vi "CommonVIs_UmlOpenVIRef.vi"(6 "ProjectNameIn":string, 8 "error in":errorcluster, 10 "ViPath/ViName":variant, 11 "AppRef":refnum<vi>) -> (0 "error out":errorcluster, 3 "vi reference":refnum<vi>, 4 "ProjectNameOut":string, 5 "AppRefOut":refnum<vi>)   [LabVIEW 2020]
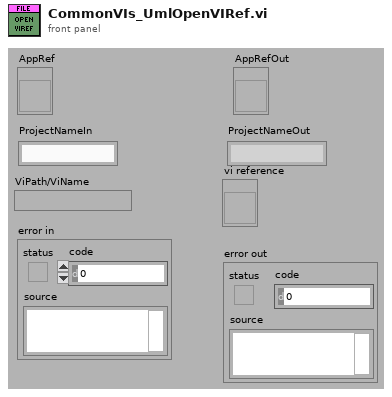
[diagram p1: front panel]
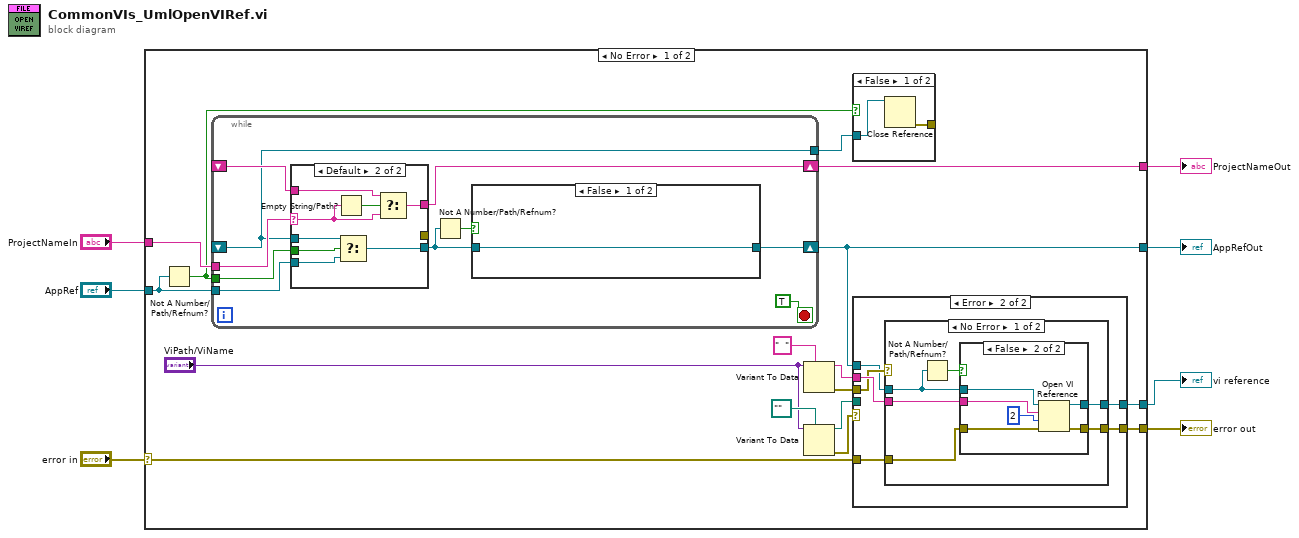
[diagram p0: block diagram]
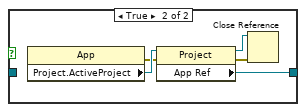
[diagram p3: hidden frame]
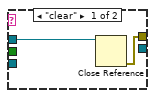
[diagram p4: hidden frame]
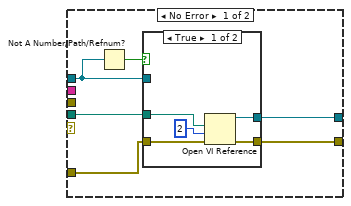
[diagram p5: hidden frame]
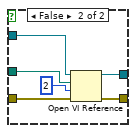
[diagram p6: hidden frame]
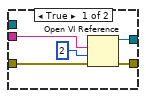
[diagram p7: hidden frame]
diagram:
  n1 = case shown="No Error" "error in" {
    selector: "error in" -> [w15 w93]
    tunnel: [w23 w93] -> w7
    tunnel: [w22 _] -> w6
    tunnel: "AppRef" -> [w10 _]
    tunnel: [w13 _] -> w3
    tunnel: "ProjectNameIn" -> [w12 _]
    tunnel: [w11 _] -> w1
    frame No Error {
      n2 = Not A Number/Path/Refnum?(number/path/refnum=w10) -> (NaN/Path/Refnum?=w9:bool)
      n3 = while {
        shift-right: [w26] -> w13
        shift-left: _ -> [w29]
        tunnel: w10 -> [w34]
        shift-right: [w32] -> w11
        shift-left: _ -> [w33]
        tunnel: w12 -> [w30]
        tunnel: w9 -> [w31]
        tunnel: [w29] -> w8
        stop <- TRUE stop-if-true
        n4 = case shown="Default" w30 {
          selector: w30 -> [_ w44]
          tunnel: w34 -> [_ w51]
          tunnel: [_ w50] -> w27
          tunnel: w33 -> [_ w49]
          tunnel: [_ w48] -> w32
          tunnel: w31 -> [_ w47]
          tunnel: w29 -> [w43 w46]
          tunnel: [w42 _] -> _
          frame "clear" {
            n5 = Close Reference(reference=w43) -> (error out=w42:errorcluster)  [unwired: 1 in]
          }
          frame Default {
            n6 = Empty String/Path?(string/path=w44) -> (empty?=w45:bool)
            n7 = Select(t=w46, s=w47, f=w51) -> (s? t:f=w50:refnum<vi>)
            n8 = Select(t=w49, s=w45, f=w44) -> (s? t:f=w48:string)
          }
        }
        n9 = Not A Number/Path/Refnum?(number/path/refnum=w27) -> (NaN/Path/Refnum?=w28:bool)
        n10 = case shown="False" w28 {
          tunnel: w27 -> [w36 _]
          tunnel: [w36 w37] -> w26
          frame False {
          }
          frame True {
            n11 = property class="App"() -> (error out=w40:errorcluster, "Project.ActiveProject"=w41:refnum<vi>)  [unwired: 2 in, 1 out]
            n12 = property class="Project"(reference=w41, error in=w40) -> (reference out=w38:refnum<vi>, error out=w39:errorcluster, "App Ref"=w37:refnum<vi>)
            n13 = Close Reference(reference=w38, error in (no error)=w39) -> ()  [unwired: 1 out]
          }
        }
      }
      n14 = Variant To Data(type="  ", Variant="ViPath/ViName") -> (data=w16:string, error out=w14:errorcluster)  [unwired: 1 in]
      n15 = Variant To Data(type=path "" ("vi path"), Variant="ViPath/ViName") -> (data=w20:path, error out=w19:errorcluster)  [unwired: 1 in]
      n16 = case shown="False" w9 {
        tunnel: w8 -> [w25 _]
        tunnel: [w24 _] -> _
        frame False {
          n17 = Close Reference(reference=w25) -> (error out=w24:errorcluster)  [unwired: 1 in]
        }
        frame True {
        }
      }
      n18 = case shown="Error" w19 {
        tunnel: w15 -> [w55 w74]
        tunnel: [w53 w73] -> w23
        tunnel: [w54 w72] -> w22
        tunnel: w20 -> [w56 _]
        tunnel: w16 -> [_ w71]
        tunnel: w14 -> [_ w70]
        tunnel: w13 -> [w52 w69]
        frame No Error {
          n19 = Not A Number/Path/Refnum?(number/path/refnum=w52) -> (NaN/Path/Refnum?=w57:bool)
          n20 = case shown="True" w57 {
            tunnel: w55 -> [w62 w68]
            tunnel: [w61 w67] -> w53
            tunnel: [w60 w66] -> w54
            tunnel: w56 -> [w59 w65]
            tunnel: w52 -> [_ w63]
            frame True {
              n21 = Open VI Reference(vi path=w59, options=2, error in (no error)=w62) -> (vi reference=w60:refnum<vi>, error out=w61:errorcluster)  [unwired: 3 out]
            }
            frame False {
              n22 = Open VI Reference(application reference (local)=w63, vi path=w65, options=2, error in (no error)=w68) -> (vi reference=w66:refnum<vi>, error out=w67:errorcluster)  [unwired: 2 out]
            }
          }
        }
        frame Error {
          n23 = case shown="No Error" w70 {
            tunnel: w74 -> [w80 w92]
            tunnel: [w79 w92] -> w73
            tunnel: [w78 _] -> w72
            tunnel: w71 -> [w77 _]
            tunnel: w69 -> [w76 _]
            frame No Error {
              n24 = Not A Number/Path/Refnum?(number/path/refnum=w76) -> (NaN/Path/Refnum?=w75:bool)
              n25 = case shown="False" w75 {
                tunnel: w80 -> [w85 w91]
                tunnel: [w84 w90] -> w79
                tunnel: [w83 w89] -> w78
                tunnel: w77 -> [w82 w88]
                tunnel: w76 -> [_ w86]
                frame True {
                  n26 = Open VI Reference(vi path=w82, options=2, error in (no error)=w85) -> (vi reference=w83:refnum<vi>, error out=w84:errorcluster)  [unwired: 3 out]
                }
                frame False {
                  n27 = Open VI Reference(application reference (local)=w86, vi path=w88, options=2, error in (no error)=w91) -> (vi reference=w89:refnum<vi>, error out=w90:errorcluster)  [unwired: 2 out]
                }
              }
            }
            frame Error {
            }
          }
        }
      }
    }
    frame Error {
    }
  }
  "vi reference" <- w6
  "error out" <- w7
  "AppRefOut" <- w3
  "ProjectNameOut" <- w1
